vi "REQ Config Std Waveform.vi"(8 "error in":errorcluster, 10 "Std Waveform Setting":T1={"Waveform Function (1: Sine)"=1, "Frequency (1000 Hz)"=1000.0, "Amplitude (1)"=1.0, "Unit (0: Vpp)"=0, "DC Offset (0.00 V)"=0.0} {"Unit (0: Vpp)" items=["Vpp", "Vrms", "dB"]; "Waveform Function (1: Sine)" items=["DC", "Sine", "Square", "Triangle", "Ramp", "Pulse", "Noise", "Sinc", "Negative Ramp", "Exponential Rise", "Exponential Fall", "Cardiac"]}) -> (0 "error out":errorcluster)   [LabVIEW 2021, in "Func Generator.lvlib"]
doc: "_____\nCreated using DQMH Event Scripter 6.1.0.128."
uses:
  Func Generator.lvlib
  REQ Config Std Waveform Argument--cluster.ctl
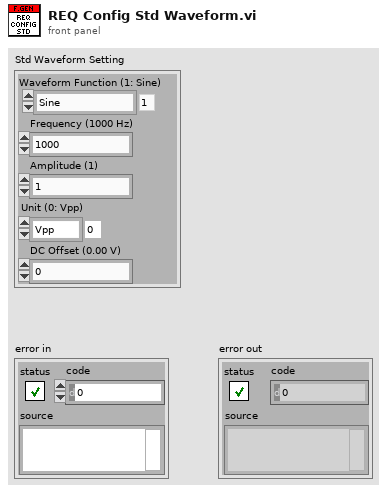
[diagram p1: front panel]
types:
  T1 = cluster{"Waveform Function (1: Sine)":u16, "Frequency (1000 Hz)":dbl, "Amplitude (1)":dbl, "Unit (0: Vpp)":u16, "DC Offset (0.00 V)":dbl}
  T2 = typedef "Func Generator.lvlib/REQ Config Std Waveform Argument--cluster.ctl" = cluster{"Std Waveform Setting":cluster{"Waveform Function (1: Sine)":u16, "Frequency (1000 Hz)":dbl, "Amplitude (1)":dbl, "Unit (0: Vpp)":u16, "DC Offset (0.00 V)":dbl}}
  T3 = typedef "Func Generator.lvlib/Request Events--cluster.ctl" = cluster{"Stop Module":refnum<user-event>, "Show Panel":refnum<user-event>, "Hide Panel":refnum<user-event>, "Get Module Execution Status":refnum<user-event>, "Show Diagram":refnum<user-event>, "REQ Initialize Hardware":refnum<user-event>, "REQ Enable Output":refnum<user-event>, "REQ Set Output Impedance":refnum<user-event>, "REQ Config Std Waveform":refnum<user-event>, "REQ Config Freq Sweep":refnum<user-event>, "REQ Self Test":refnum<user-event>, "REQ Close Ref":refnum<user-event>}
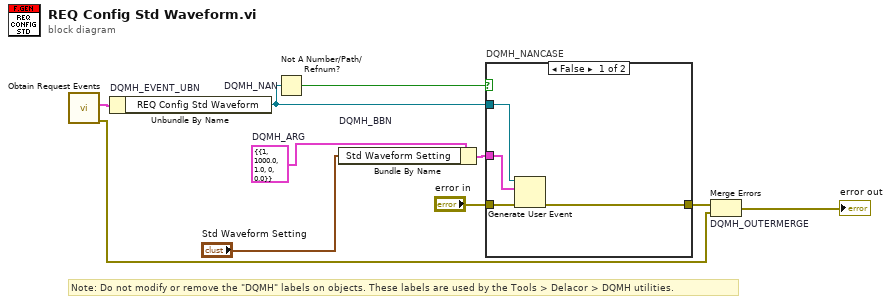
[diagram p0: block diagram]
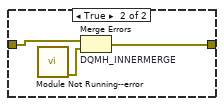
[diagram p2: hidden frame]
diagram:
  w4 = T2 {"Std Waveform Setting"={"Waveform Function (1: Sine)"=1, "Frequency (1000 Hz)"=1000.0, "Amplitude (1)"=1.0, "Unit (0: Vpp)"=0, "DC Offset (0.00 V)"=0.0}}  # DQMH_ARG
  # "Note: Do not modify or remove the \"DQMH\" labels on objects. These labels are used by the Tools > Delacor > DQMH utilities."
  n1 = call "Obtain Request Events.vi"() -> ("error out"=w2:errorcluster, "Func Generator Request Events"=w1:T3)  [unwired: 10 in]
  n2 = Unbundle By Name "DQMH_EVENT_UBN"(w1) -> ("REQ Config Std Waveform"=w6:refnum<user-event>)
  n3 = Not A Number/Path/Refnum? "DQMH_NAN"(number/path/refnum=w6) -> (NaN/Path/Refnum?=w7:bool)
  n4 = Bundle By Name "DQMH_BBN"(cluster=w4, "Std Waveform Setting"="Std Waveform Setting") -> (w8:T2)
  n5 = case "DQMH_NANCASE" shown="False" w7 {
    tunnel: "error in" -> [w14 w17]
    tunnel: [w13 w16] -> w5
    tunnel: w6 -> [w12 _]
    tunnel: w8 -> [w11 _]
    frame False {
      n6 = Generate User Event(user event=w12, event data cluster=w11, error in=w14) -> (error out=w13:errorcluster)  [unwired: 1 in, 1 out]
    }
    frame True {
      n7 = call "Module Not Running--error.vi"() -> ("error out"=w15:errorcluster)  [unwired: 11 in]
      n8 = Merge Errors "DQMH_INNERMERGE"(w17, w15) -> (w16:errorcluster)
    }
  }
  n9 = Merge Errors "DQMH_OUTERMERGE"(w5, w2) -> (→"error out":errorcluster)
